vi "Generic Section.vi"(8 "error in (no error)":errorcluster, 11 "Node Ptr":T1 format="%.0x") -> (0 "error out":errorcluster)   [LabVIEW 2019, in "Profile Interpolation System Explorer.lvlib"]
uses:
  Profile Interpolation System Explorer.lvlib
  <vilib>/NI VeriStand/Custom Device API/Custom Device Item Ref.ctl
  <vilib>/NI VeriStand/Custom Device API/Custom Device API.lvlib
panel:
  in  "SHDocVw.IWebBrowser":refnum<k7>(container)
  in  "Specific Header":cluster{"Section Name":string}={"Section Name"="Specific Page Settings"}
  in  "General Header":cluster{"Section Name":string}={"Section Name"="General Page Settings"}
  in  "Description":string
  out "Name":string
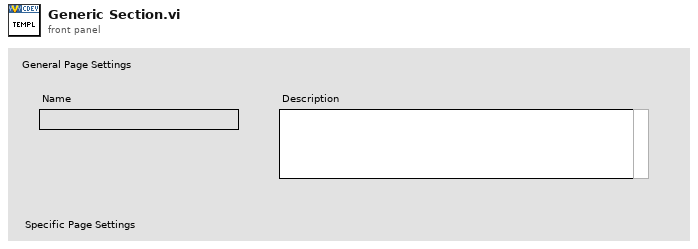
[diagram p1: front panel]
types:
  T1 = typedef "Custom Device API.lvlib/Custom Device Item Ref.ctl" = u64
  T2 = typedef "Custom Device API.lvlib/Custom Device Item Info.ctl" = cluster{"Name":string, "Is Channel":bool, "GUID":string, "Is Waveform":bool}
  T3 = typedef "Custom Device API.lvlib/Custom Device Commands.ctl" = enum16{"Default", "Item renamed", "Shutdown", "Dynamic button pressed"}
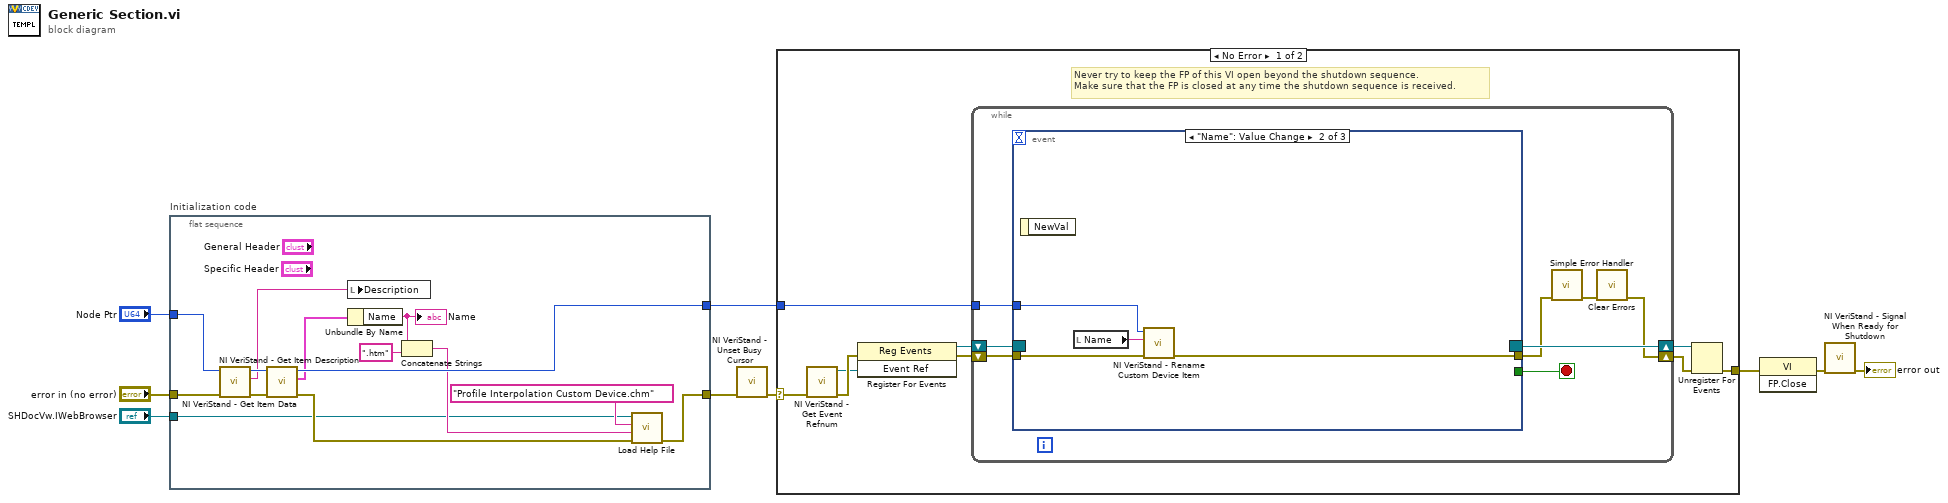
[diagram p0: block diagram]
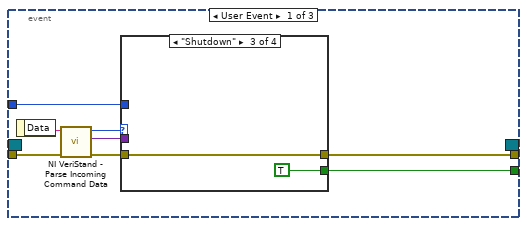
[diagram p2: hidden frame]
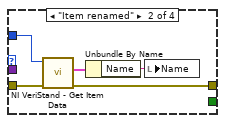
[diagram p4: hidden frame]
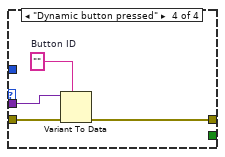
[diagram p5: hidden frame]
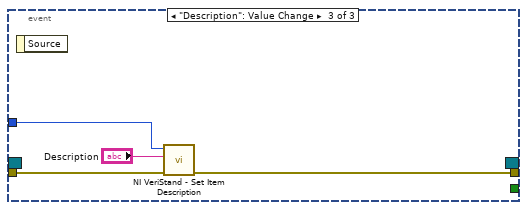
[diagram p6: hidden frame]
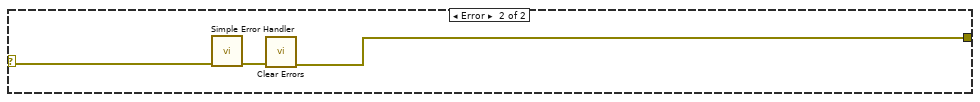
[diagram p7: hidden frame]
diagram:
  n1 = flat-sequence "Initialization code" {
    tunnel: "error in (no error)" -> [w10]
    tunnel: "Node Ptr" -> [w19]
    tunnel: [w14] -> w5
    tunnel: [w23] -> w2
    tunnel: "SHDocVw.IWebBrowser" -> [w11]
    frame #0 {
      n2 = call <vilib>:"NI VeriStand - Get Item Description.vi"("error in (no error)"=w10, "Item Ref in"=w19) -> ("error out"=w21:errorcluster, "Description"=w18:string, "Item Ref out"=w22:T1)  [unwired: 7 out]
      n3 = call <vilib>:"NI VeriStand - Get Item Data.vi"("error in (no error)"=w21, "Item Ref in"=w22) -> ("error out"=w15:errorcluster, "Item Info"=w20:T2, "Item Ref out"=w23:T1)  [unwired: 7 out]
      n4 = local write "Description"(w18) -> ()
      n5 = Unbundle By Name(w20) -> ("Name"=w17:string)
      "Name" <- w17
      n6 = Concatenate Strings(w17, ".htm" ("string")) -> (w13:string)
      n7 = call "Load Help File.vi"("error in (no error)"=w15, "HTML File"=w13, "Main CHM File"="Profile Interpolation Custom Device.chm" ("CD_CHM_FileName"), "SHDocVw.IWebBrowser2"=w11) -> ("error out"=w14:errorcluster)  [unwired: 7 in]
    }
  }
  n8 = call <vilib>:"NI VeriStand - Unset Busy Cursor.vi"("error in (no error)"=w5) -> ("error out"=w4:errorcluster)  [unwired: 10 out]
  n9 = case shown="No Error" w4 {
    selector: w4 -> [w24 w71]
    tunnel: [w29 w69] -> w9
    tunnel: w2 -> [w25 _]
    frame No Error {
      # "Never try to keep the FP of this VI open beyond the shutdown sequence.\nMake sure that the FP is closed at any time the shutdown sequence is received."
      n10 = call <vilib>:"NI VeriStand - Get Event Refnum.vi"("error in (no error)"=w24) -> ("error out"=w32:errorcluster, "Event Ref"=w28:refnum<user-event>)  [unwired: 9 out]
      n11 = register-events(error in=w32, w28) -> (reference out=w26:refnum<event-registration>, error out=w27:errorcluster)  [unwired: 1 in]
      n12 = while {
        tunnel: w25 -> [w36]
        shift-right: [w33] -> w30
        shift-left: w27 -> [w39]
        shift-right: [w40] -> w31
        shift-left: w26 -> [w38]
        stop <- w37 stop-if-true
        n13 = event shown="[1] \"Name\": Value Change" {
          selector: w38 -> [_ _ _]
          dyn-events: [_ _ _] -> w40
          timeout: _ -> [_ _ _]
          tunnel: w39 -> [w48 w64 w67]
          tunnel: [w44 _ _] -> w37
          tunnel: [w43 w63 w66] -> w35
          tunnel: w36 -> [w42 w62 w68]
          event User Event {
            n14 = event-data() -> ("Data"=w47:string)  [unwired: 1 out]
            n15 = call <vilib>:"NI VeriStand - Parse Incoming Command Data.vi"("error in (no error)"=w48, "Incoming data"=w47) -> ("error out"=w46:errorcluster, "Outgoing data"=w41:variant, "Action"=w45:T3)  [unwired: 7 out]
            n16 = case shown="\"Shutdown\"" w45 {
              tunnel: w46 -> [w49 w54 w55 w60]
              tunnel: [_ _ TRUE _] -> w44
              tunnel: [w49 w51 w55 w57] -> w43
              tunnel: w42 -> [_ w53 _ _]
              tunnel: w41 -> [_ _ _ w59]
              frame "Default", Default {
              }
              frame "Item renamed" {
                n17 = call <vilib>:"NI VeriStand - Get Item Data.vi"("error in (no error)"=w54, "Item Ref in"=w53) -> ("error out"=w51:errorcluster, "Item Info"=w52:T2)  [unwired: 8 out]
                n18 = Unbundle By Name(w52) -> ("Name"=w50:string)
                n19 = local write "Name"(w50) -> ()
              }
              frame "Shutdown" {
              }
              frame "Dynamic button pressed" {
                w58 = ""  # Button ID
                n20 = Variant To Data(error in=w60, type=w58, Variant=w59) -> (error out=w57:errorcluster)  [unwired: 1 out]
              }
            }
          }
          event "Name": Value Change {
            n21 = event-data() -> ()  [unwired: 2 out]
            n22 = local read "Name"() -> (w61:string)
            n23 = call <vilib>:"NI VeriStand - Rename Custom Device Item.vi"("error in (no error)"=w64, "New Name"=w61, "Item Ref in"=w62) -> ("error out"=w63:errorcluster)  [unwired: 1 in, 7 out]
          }
          event "Description": Value Change {
            n24 = event-data() -> ()  [unwired: 2 out]
            n25 = call <vilib>:"NI VeriStand - Set Item Description.vi"("error in (no error)"=w67, "Description"="Description", "Item Ref in"=w68) -> ("error out"=w66:errorcluster)  [unwired: 8 out]
          }
        }
        n26 = call <vilib>:"Simple Error Handler.vi"("error in (no error)"=w35) -> ("error out"=w34:errorcluster)  [unwired: 1 in, 7 out]
        n27 = call <vilib>:"Clear Errors.vi"("error in (no error)"=w34) -> ("error out"=w33:errorcluster)  [unwired: 1 in, 5 out]
      }
      n28 = Unregister For Events(event registration refnum=w31, error in=w30) -> (error out=w29:errorcluster)
    }
    frame Error {
      n29 = call <vilib>:"Simple Error Handler.vi"("error in (no error)"=w71) -> ("error out"=w70:errorcluster)  [unwired: 1 in, 7 out]
      n30 = call <vilib>:"Clear Errors.vi"("error in (no error)"=w70) -> ("error out"=w69:errorcluster)  [unwired: 1 in, 5 out]
    }
  }
  n31 = invoke class="VI" method="FP.Close"(error in=w9) -> (error out=w8:errorcluster)  [unwired: 2 in, 2 out]
  n32 = call <vilib>:"NI VeriStand - Signal When Ready for Shutdown.vi"("error in (no error)"=w8) -> ("error out"=→"error out":errorcluster)  [unwired: 10 out]
